vi "Reply.vi"(7 "Reply":T1, 8 "error in (no error)":errorcluster, 11 "ReplyPayload":variant) -> (0 "error out":errorcluster)   [LabVIEW 2024, in "Module.lvclass"]
uses:
  Module.lvclass
  Module.lvclass/Module.ctl
  Reply.ctl
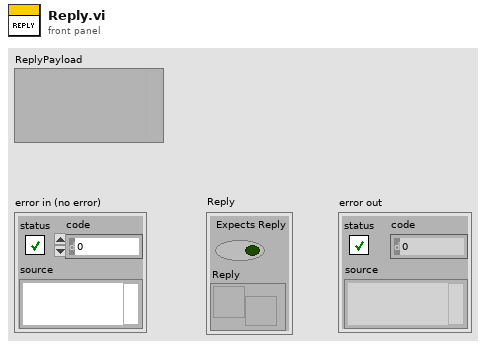
[diagram p1: front panel]
types:
  T1 = typedef "Module.lvclass/Reply.ctl" = cluster{"Expects Reply":bool, "Reply":refnum<notifier>}
  T2 = cluster{"ReplyPayload":variant, "error in (no error)":errorcluster}
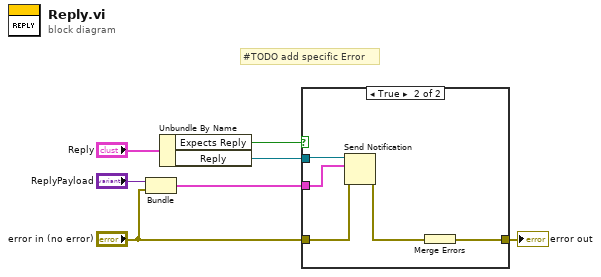
[diagram p0: block diagram]
diagram:
  # "#TODO add specific Error"
  n1 = Bundle("ReplyPayload"="ReplyPayload", "error in (no error)"="error in (no error)") -> (w2:T2)  [unwired: 1 in]
  n2 = Unbundle By Name("Reply") -> ("Expects Reply"=w6:bool, "Reply"=w5:refnum<notifier>)
  n3 = case shown="True" w6 {
    tunnel: w5 -> [_ w13]
    tunnel: [w8 w11] -> w4
    tunnel: w2 -> [_ w12]
    tunnel: "error in (no error)" -> [w8 w9]
    frame False {
    }
    frame True {
      n4 = Send Notification(notification=w12, notifier=w13, error in (no error)=w9) -> (error out=w10:errorcluster)  [unwired: 1 out]
      n5 = Merge Errors(w10) -> (w11:errorcluster)
    }
  }
  "error out" <- w4
